vi "Get runtime chain.vi"() -> ()   [LabVIEW 2012, in "DAQCascade512.lvclass"]
uses:
  DAQCascade512.lvclass
  DAQCascade512.lvclass/DAQCascade512.ctl
panel:
  out "runtime chain":variant[](array[variant])
  out "Cascade512Base out":refnum<class "DAQCascade512.lvclass">
  in  "Cascade512Base in":refnum<class "DAQCascade512.lvclass">
  out "error out":errorcluster
  in  "error in (no error)":errorcluster
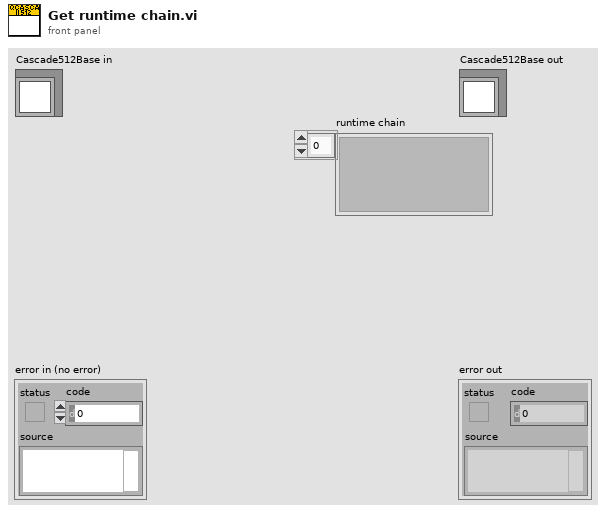
[diagram p1: front panel]
types:
  T1 = typedef "DAQCascade512.lvclass/runtime cluster.ctl" = cluster{"Camera Handle":u32, "Image Handle":u32, "Xdim":u32, "Ydim":u32}
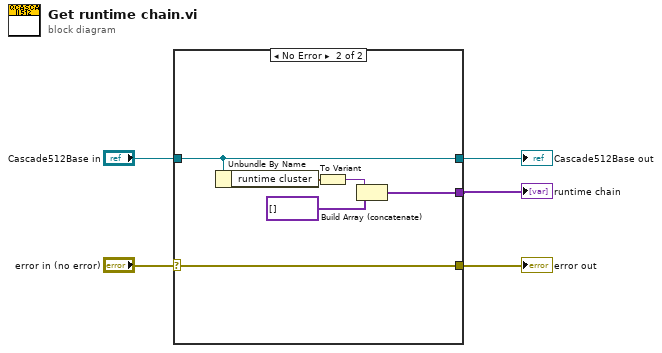
[diagram p0: block diagram]
diagram:
  n1 = case shown="No Error" "error in (no error)" {
    selector: "error in (no error)" -> [w6 w10]
    tunnel: "Cascade512Base in" -> [w7 w13]
    tunnel: [w7 w13] -> w5
    tunnel: [_ w8] -> w1
    tunnel: [w6 w10] -> w4
    frame Error {
    }
    frame No Error {
      n2 = Unbundle By Name(w13) -> ("runtime cluster"=w12:T1)
      n3 = To Variant(anything=w12) -> (Variant=w11:variant)
      n4 = Build Array (concatenate)(w11, variant[] [] ("array")) -> (w8:variant[])
    }
  }
  "error out" <- w4
  "Cascade512Base out" <- w5
  "runtime chain" <- w1
